vi "rvc 2D Euler to Homogeneous (vector).vi"(8 "error in (no error)":errorcluster, 11 "Euler":dbl[](array[numeric])) -> (0 "Error Out":errorcluster, 3 "Homogeneous":T1)   [LabVIEW 2013]
uses:
  <vilib>/Analysis/Matrix/Datatypes/RealMatrix.ctl
  <vilib>/Analysis/Matrix/NI_Matrix.lvlib
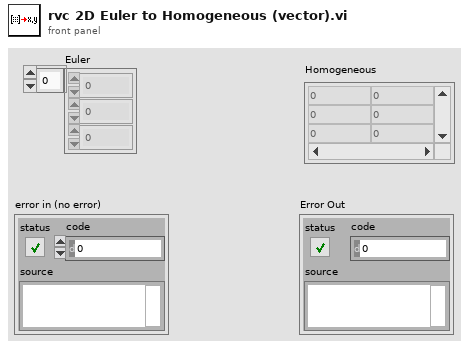
[diagram p1: front panel]
types:
  T1 = typedef "NI_Matrix.lvlib/RealMatrix.ctl" = dbl[][]
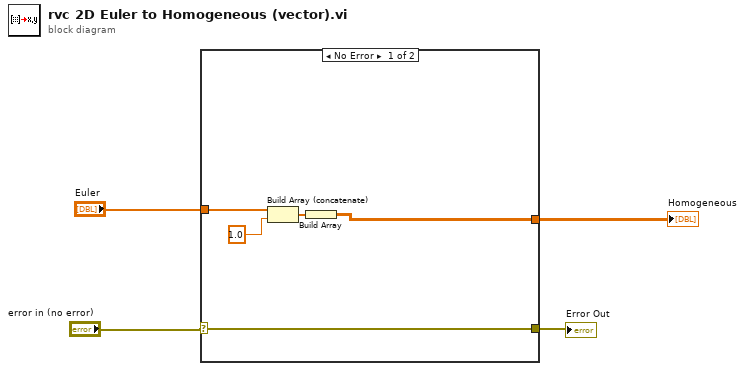
[diagram p0: block diagram]
diagram:
  n1 = case shown="No Error" "error in (no error)" {
    selector: "error in (no error)" -> [w9 w10]
    tunnel: [w9 w10] -> w4
    tunnel: "Euler" -> [w8 _]
    tunnel: [w5 _] -> w1
    frame No Error {
      n2 = Build Array (concatenate)(w8, 1.0) -> (w6:dbl[])
      n3 = Build Array(w6) -> (w5:T1)
    }
    frame Error {
    }
  }
  "Error Out" <- w4
  "Homogeneous" <- w1
